vi "Dpc Get Tdo Bits.vi"(0 "hif":u32, 1 "rgbRcv":string, 2 "ptrid":u16, 5 "cbits":i32, 7 "bitTdi":i32, 9 "bitTms":i32, 11 "error in (no error)":errorcluster, 12 "perc":i32) -> (3 "rgbRcv out":string, 4 "hif out":u32, 6 "ptrid out":u16, 8 "function return":i32, 14 "perc out":i32, 15 "error out":errorcluster)   [LabVIEW 2011, in "LVH-Adept.lvlib" / "DPCUTIL.lvlib"]
doc: "DPCAPI BOOL DpcGetTdoBits(HANDLE hif, INT32 cbits, BOOL bitTdi, BOOL bitTms, BYTE *rgbRcv, ERC *perc, TRID *ptrid);"
uses:
  DPCUTIL.lvlib
  Resources/dpcutil.dll
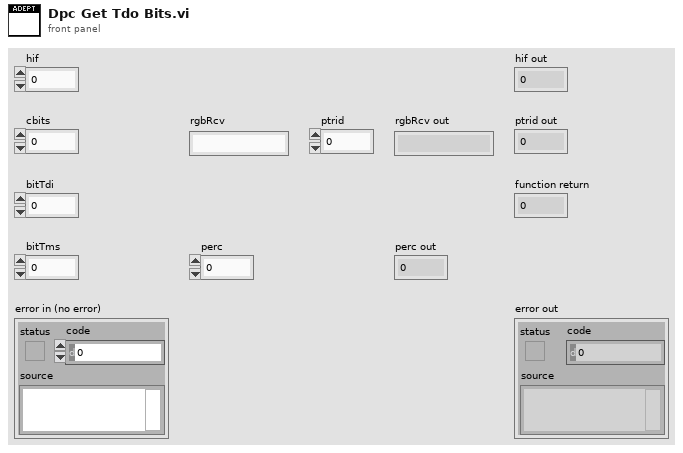
[diagram p1: front panel]
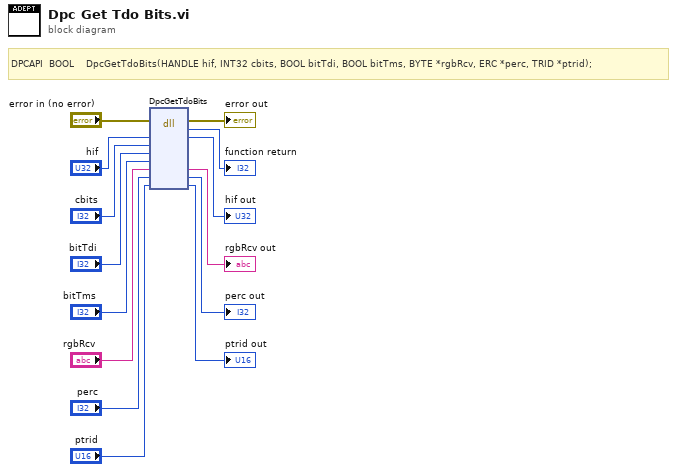
[diagram p0: block diagram]
diagram:
  # "DPCAPI  BOOL    DpcGetTdoBits(HANDLE hif, INT32 cbits, BOOL bitTdi, BOOL bitTms, BYTE *rgbRcv, ERC *perc, TRID *ptrid);"
  n1 = dll-call lib="C:/github/labviewhacker/LVH-Adept/LabVIEW/vi.lib/LabVIEW Hacker/Adept/Private/Resources/dpcutil.*" fn="DpcGetTdoBits"(error in="error in (no error)", "hif"="hif", "cbits"="cbits", "bitTdi"="bitTdi", "bitTms"="bitTms", "rgbRcv"="rgbRcv", "perc"="perc", "ptrid"="ptrid") -> (error out=→"error out":errorcluster, →"function return":i32, "hif"=→"hif out":u32, "rgbRcv"=→"rgbRcv out":string, "perc"=→"perc out":i32, "ptrid"=→"ptrid out":u16)  [unwired: 5 in, 1 out]
